vi "PID_controller_17.vi"() -> ()   [LabVIEW 2011]
panel:
  in  "Local":bool
  in  "Hold":bool
  out "tune_Method":u16(ring) items=["Setpoint", "Angle"]
  in  "Method":u16(ring)=1 items=["Setpoint", "Angle"]
  in  "Setpoint":u16(ring)=2 items=["A", "B", "C", "D"]
  out "do_tune":bool
  in  "Tune":bool
  out "Tune Set Point (torr)":dbl format="%.2f"
  in  "stop":bool
  out "fit":cluster{"element":dbl, "Value":dbl}[](array[cluster])
  out "err_avg":dbl
  out "Setpoint":string
  in  "Ks":dbl
  out "dt(s)":dbl
  out "windup error":dbl
  out "tPrev":dbl
  out "target value":dbl
  out "error(t-t0)":cluster{dbl, "Value":dbl}[](array[cluster])
  out "error":dbl
  out "tStart(s)":dbl
  out "S00":dbl
  out "S10":dbl
  out "S20":dbl
  out "S11":dbl
  out "S01":dbl
  out "weight":dbl[](array[numeric])
  in  "# of points to watch":i32=60
  in  "tSmooth(s)":dbl=4.0
  out "t0":dbl
  out "error(t)":cluster{dbl, "Value":dbl}[](array[cluster])
  out "error out":errorcluster
  out "first":bool=TRUE
  out "XY Graph":T1(graph)
  out "current value":dbl
  in  "Period (s)":dbl=1.0
  out "dValue":dbl
  out "derivative":dbl
  out "integral":dbl
  out "Angle (deg)":dbl format="%#.1f"
  in  "Kd":dbl=0.4
  in  "Ki":dbl
  in  "Kp":dbl=-0.1
  out "Current P (torr)":dbl format="%.2f"
  in  "Set Point (torr)":dbl format="%.2f"
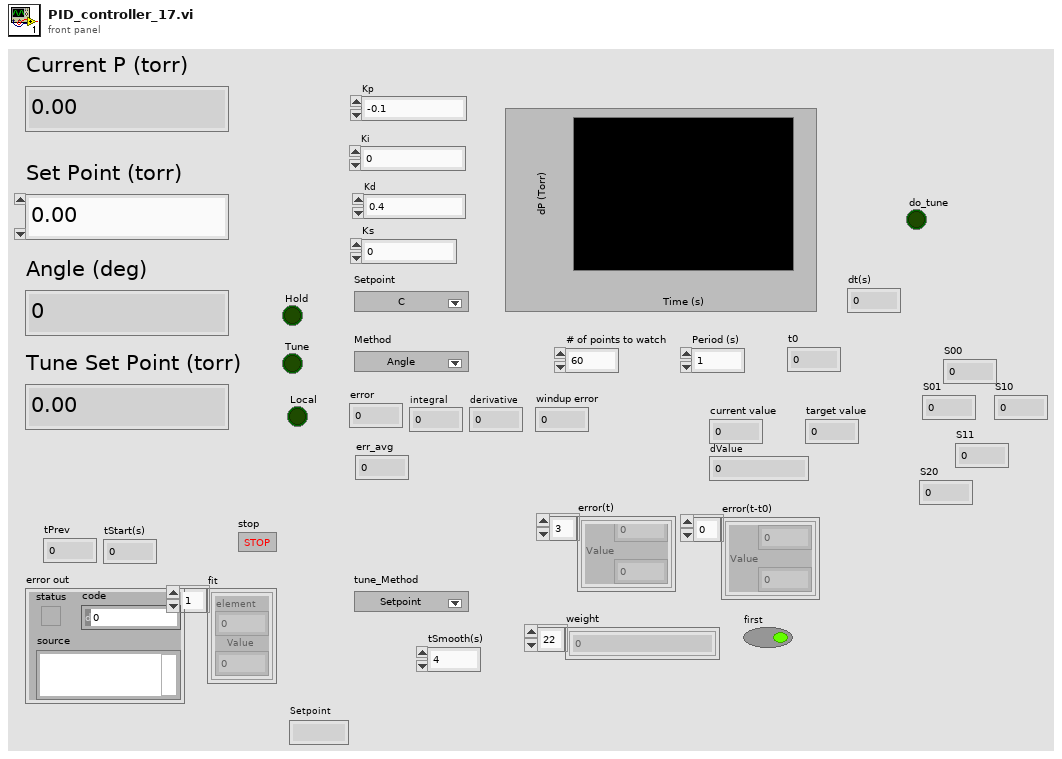
[diagram p1: front panel]
types:
  T1 = cluster{"Value":cluster{"element":dbl, "Value":dbl}[]}[]
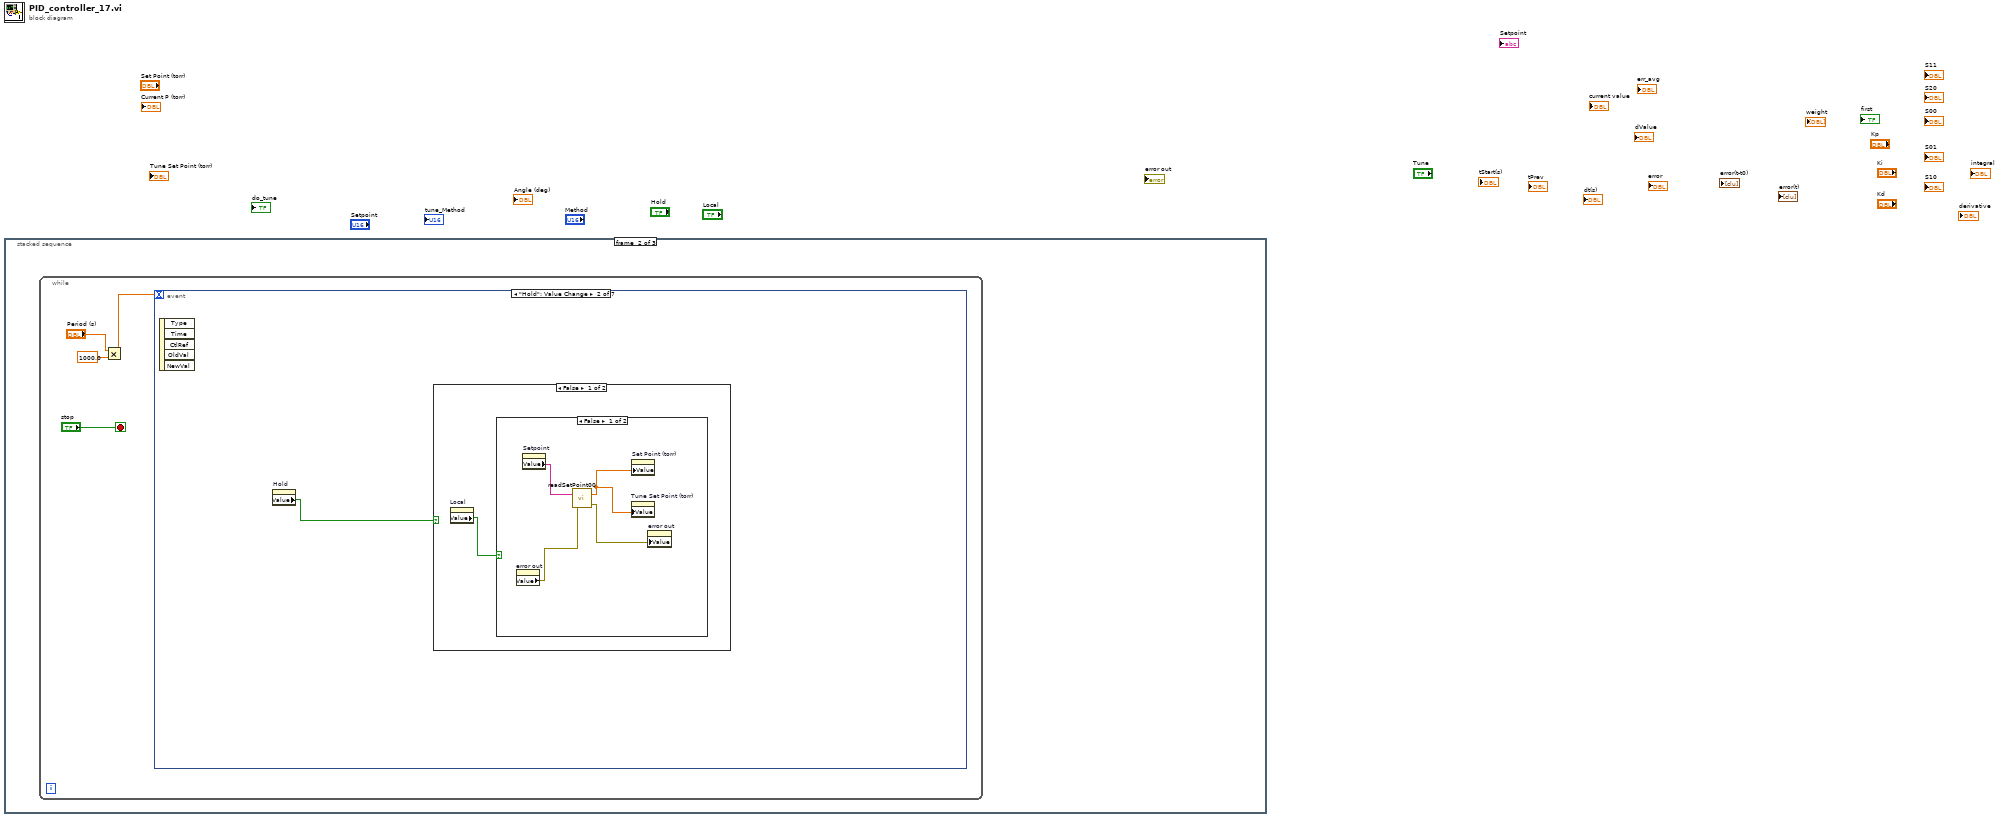
[diagram p0: block diagram]
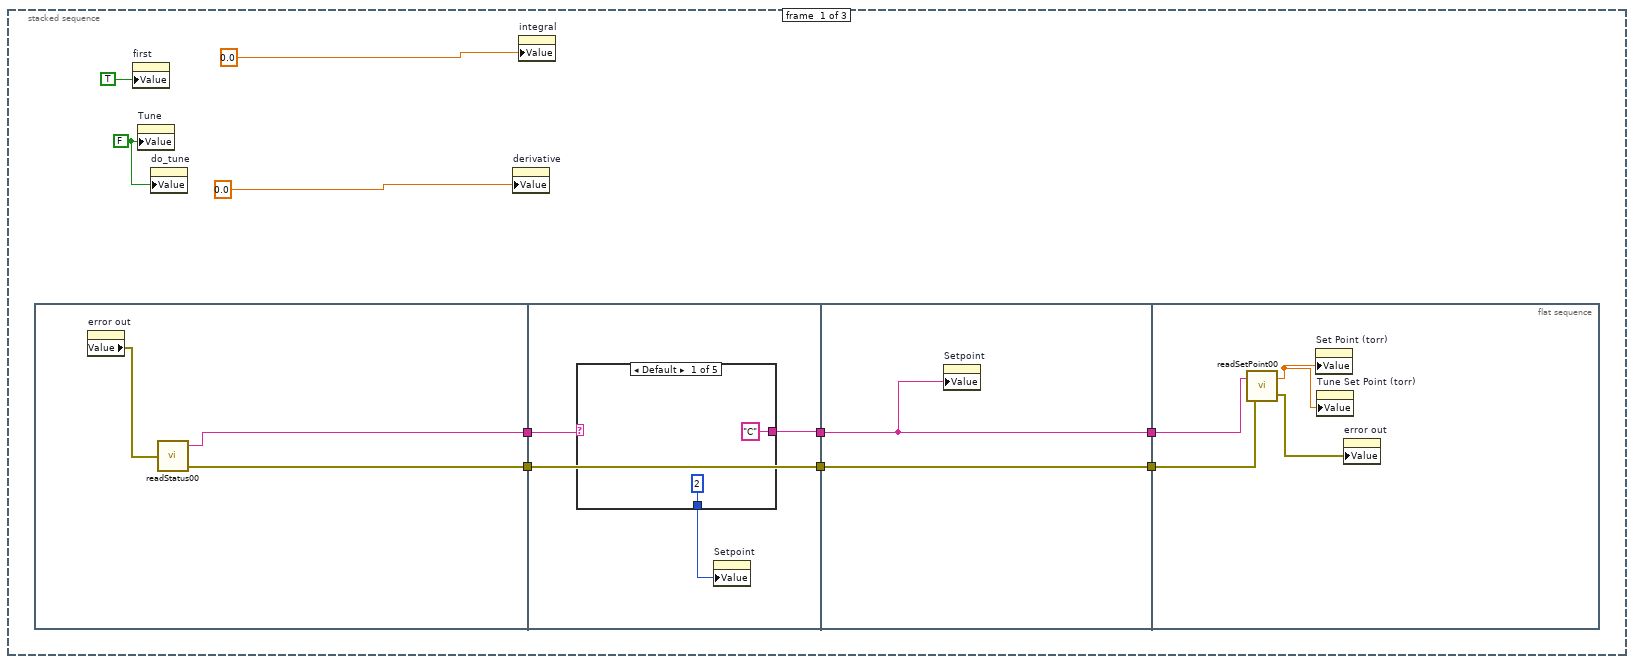
[diagram p2: hidden frame]
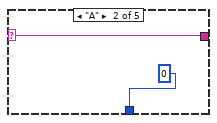
[diagram p3: hidden frame]
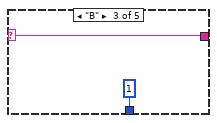
[diagram p4: hidden frame]
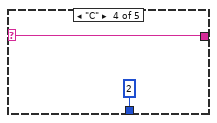
[diagram p5: hidden frame]
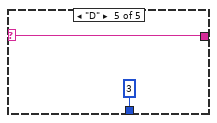
[diagram p6: hidden frame]
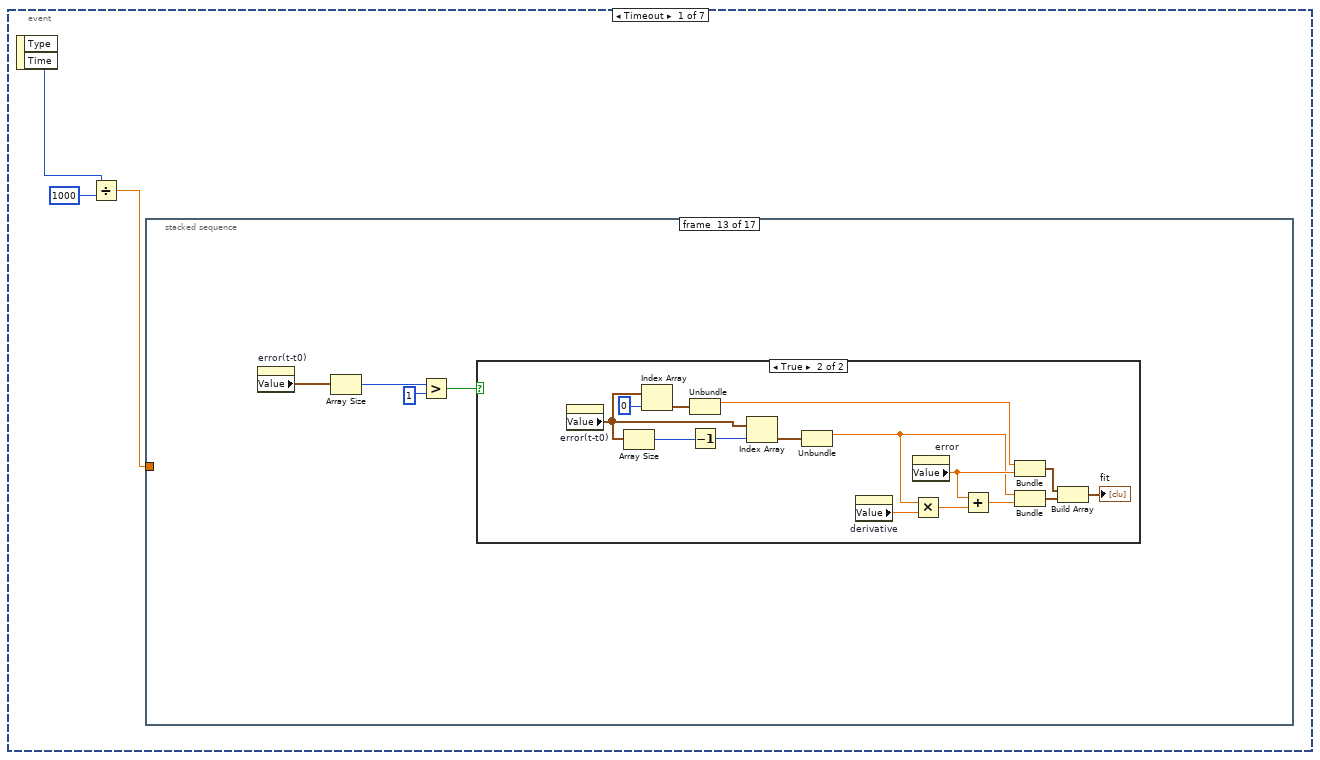
[diagram p7: hidden frame]
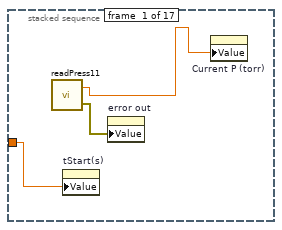
[diagram p8: hidden frame]
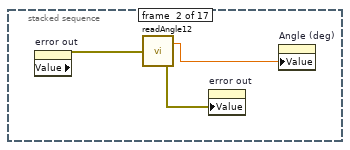
[diagram p9: hidden frame]
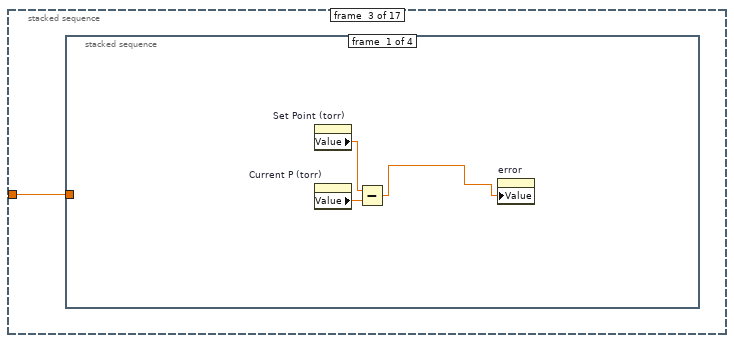
[diagram p10: hidden frame]
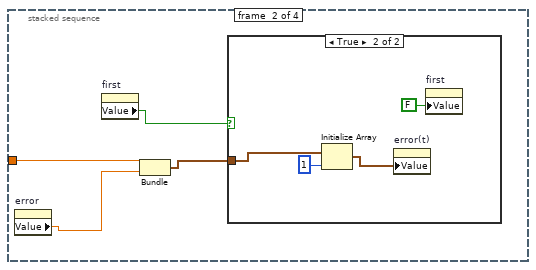
[diagram p11: hidden frame]
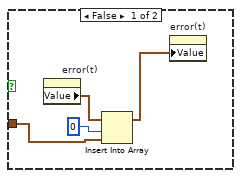
[diagram p12: hidden frame]
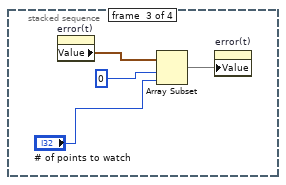
[diagram p13: hidden frame]
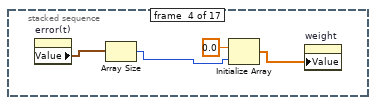
[diagram p15: hidden frame]
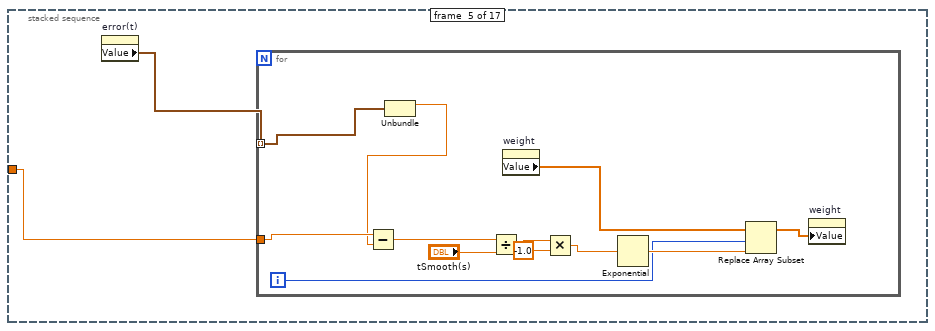
[diagram p16: hidden frame]
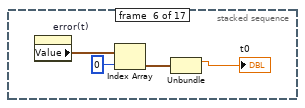
[diagram p17: hidden frame]
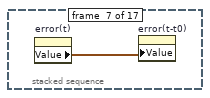
[diagram p18: hidden frame]
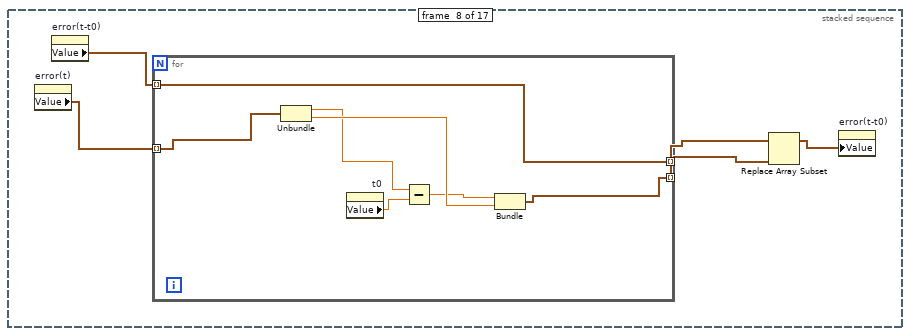
[diagram p19: hidden frame]
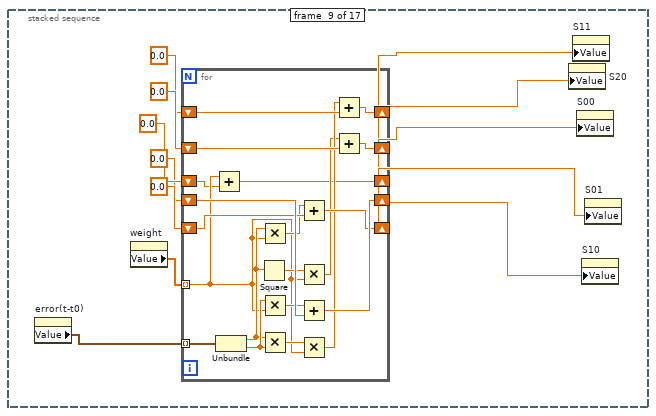
[diagram p20: hidden frame]
diagram:
  n1 = stacked-sequence {
    frame #0 {
      w7 = FALSE ("Tune")
      n2 = flat-sequence {
        tunnel: [w12] -> w6
        tunnel: [w11] -> w5
        tunnel: w6 -> [w16]
        tunnel: [w15] -> w4
        tunnel: w5 -> [w17]
        tunnel: [w17] -> w2
        tunnel: w4 -> [w28]
        tunnel: [w28] -> w3
        tunnel: w2 -> [w29]
        tunnel: [w29] -> w1
        tunnel: w3 -> [w33]
        tunnel: w1 -> [w32]
        frame #0 {
          n3 = property on="error out" class="Clust (strict)"() -> ("Value"=w13:errorcluster)  [unwired: 2 in, 2 out]
          n4 = call "readStatus00.vi"("error in"=w13) -> ("Setpoint"=w12:string, "error out"=w11:errorcluster)  [unwired: 1 out]
        }
        frame #1 {
          n5 = case shown="Default" w16 {
            selector: w16 -> [_ w21 w22 w24 w26]
            tunnel: ["C" w21 w22 w24 w26] -> w15
            tunnel: [u16 2 ("Ring") u16 0 ("Ring") u16 1 ("Ring") u16 2 ("Ring") u16 3 ("Ring")] -> w14
            frame Default {
            }
            frame "A" {
            }
            frame "B" {
            }
            frame "C" {
            }
            frame "D" {
            }
          }
          n6 = property on="Setpoint" class="Ring (strict)"("Value"=w14) -> ()  [unwired: 2 in, 2 out]
        }
        frame #2 {
          n7 = property on="Setpoint" class="Str"("Value"=w28) -> ()  [unwired: 2 in, 2 out]
        }
        frame #3 {
          n8 = call "readSetPoint00.vi"("error in"=w32, "Setpoint"=w33) -> ("error out"=w31:errorcluster, "P"=w30:dbl)
          n9 = property on="Set Point (torr)" class="DigNum (strict)"("Value"=w30) -> ()  [unwired: 2 in, 2 out]
          n10 = property on="Tune Set Point (torr)" class="DigNum (strict)"("Value"=w30) -> ()  [unwired: 2 in, 2 out]
          n11 = property on="error out" class="Clust (strict)"("Value"=w31) -> ()  [unwired: 2 in, 2 out]
        }
      }
      n12 = property on="first" class="Bool (strict)"("Value"=TRUE ("first")) -> ()  [unwired: 2 in, 2 out]
      n13 = property on="Tune" class="Bool (strict)"("Value"=w7) -> ()  [unwired: 2 in, 2 out]
      n14 = property on="do_tune" class="Bool (strict)"("Value"=w7) -> ()  [unwired: 2 in, 2 out]
      n15 = property on="derivative" class="DigNum (strict)"("Value"=0.0 ("derivative")) -> ()  [unwired: 2 in, 2 out]
      n16 = property on="integral" class="DigNum (strict)"("Value"=0.0 ("integral")) -> ()  [unwired: 2 in, 2 out]
    }
    frame #1 {
      n17 = while {
        stop <- "stop" stop-if-true
        n18 = Multiply(x="Period (s)", y=1000.0) -> (x*y=w35:dbl)
        n19 = event shown="[1] \"Hold\": Value Change" {
          selector: _ -> [_ _ _ _ _ _ _]
          dyn-events: _ -> [_ _ _ _ _ _ _]
          timeout: w35 -> [_ _ _ _ _ _ _]
          event Timeout {
            n20 = event-data() -> ("Time"=w40:u32)  [unwired: 1 in, 1 out]
            n21 = Divide(x=w40, y=u32 1000) -> (x/y=w38:dbl)
            n22 = stacked-sequence {
              tunnel: w38 -> [w41 _ w47 _ w71 _ _ _ _ _ _ _ _ _ _ _ _]
              frame #0 {
                n23 = call "readPress11.vi"() -> ("P"=w43:dbl, "error out"=w42:errorcluster)  [unwired: 1 in]
                n24 = property on="tStart(s)" class="DigNum (strict)"("Value"=w41) -> ()  [unwired: 2 in, 2 out]
                n25 = property on="error out" class="Clust (strict)"("Value"=w42) -> ()  [unwired: 2 in, 2 out]
                n26 = property on="Current P (torr)" class="DigNum (strict)"("Value"=w43) -> ()  [unwired: 2 in, 2 out]
              }
              frame #1 {
                n27 = property on="error out" class="Clust (strict)"() -> ("Value"=w45:errorcluster)  [unwired: 2 in, 2 out]
                n28 = call "readAngle12.vi"("error in"=w45) -> ("angle"=w46:dbl, "error out"=w44:errorcluster)
                n29 = property on="error out" class="Clust (strict)"("Value"=w44) -> ()  [unwired: 2 in, 2 out]
                n30 = property on="Angle (deg)" class="DigNum (strict)"("Value"=w46) -> ()  [unwired: 2 in, 2 out]
              }
              frame #2 {
                n31 = stacked-sequence {
                  tunnel: w47 -> [_ w53 _ _]
                  frame #0 {
                    n32 = property on="Set Point (torr)" class="DigNum (strict)"() -> ("Value"=w49:dbl)  [unwired: 2 in, 2 out]
                    n33 = property on="Current P (torr)" class="DigNum (strict)"() -> ("Value"=w50:dbl)  [unwired: 2 in, 2 out]
                    n34 = Subtract(x=w49, y=w50) -> (x-y=w48:dbl)
                    n35 = property on="error" class="DigNum (strict)"("Value"=w48) -> ()  [unwired: 2 in, 2 out]
                  }
                  frame #1 {
                    n36 = property on="error" class="DigNum (strict)"() -> ("Value"=w51:dbl)  [unwired: 2 in, 2 out]
                    n37 = property on="first" class="Bool (strict)"() -> ("Value"=w54:bool)  [unwired: 2 in, 2 out]
                    n38 = Bundle(w53, "Value"=w51) -> (w52:cluster{dbl, "Value":dbl})  [unwired: 1 in]
                    n39 = case shown="True" w54 {
                      tunnel: w52 -> [w56 w61]
                      frame False {
                        n40 = property on="error(t)" class="Arr (strict)"() -> ("Value"=w57:cluster{dbl, "Value":dbl}[])  [unwired: 2 in, 2 out]
                        n41 = Insert Into Array(array=w57, index=0, new element=w56) -> (w55:cluster{dbl, "Value":dbl}[])
                        n42 = property on="error(t)" class="Arr (strict)"("Value"=w55) -> ()  [unwired: 2 in, 2 out]
                      }
                      frame True {
                        n43 = Initialize Array(w61, 1 ("dimension size")) -> (w59:cluster{dbl, "Value":dbl}[])
                        n44 = property on="error(t)" class="Arr (strict)"("Value"=w59) -> ()  [unwired: 2 in, 2 out]
                        n45 = property on="first" class="Bool (strict)"("Value"=FALSE ("first")) -> ()  [unwired: 2 in, 2 out]
                      }
                    }
                  }
                  frame #2 {
                    n46 = property on="error(t)" class="Arr (strict)"() -> ("Value"=w64:cluster{dbl, "Value":dbl}[])  [unwired: 2 in, 2 out]
                    n47 = Array Subset(array=w64, index=0, length="# of points to watch") -> (w66:cluster{dbl, "Value":dbl}[])
                    n48 = property on="error(t)" class="Arr (strict)"("Value"=w66) -> ()  [unwired: 2 in, 2 out]
                  }
                  frame #3 {
                  }
                }
              }
              frame #3 {
                n49 = property on="error(t)" class="Arr (strict)"() -> ("Value"=w67:cluster{dbl, "Value":dbl}[])  [unwired: 2 in, 2 out]
                n50 = Array Size(array=w67) -> (size(s)=w69:i32)
                n51 = Initialize Array(0.0 ("element"), w69) -> (w70:dbl[])
                n52 = property on="weight" class="Arr (strict)"("Value"=w70) -> ()  [unwired: 2 in, 2 out]
              }
              frame #4 {
                n53 = property on="error(t)" class="Arr (strict)"() -> ("Value"=w72:cluster{dbl, "Value":dbl}[])  [unwired: 2 in, 2 out]
                n54 = for {
                  tunnel: w72 -> [w84] mode=indexing
                  tunnel: w71 -> [w83]
                  i -> [w79]
                  n55 = Unbundle(w84) -> (w82:dbl)  [unwired: 1 out]
                  n56 = Subtract(x=w83, y=w82) -> (x-y=w77:dbl)
                  n57 = Divide(x=w77, y="tSmooth(s)") -> (x/y=w75:dbl)
                  n58 = property on="weight" class="Arr (strict)"() -> ("Value"=w80:dbl[])  [unwired: 2 in, 2 out]
                  n59 = Multiply(x=w75, y=-1.0) -> (x*y=w73:dbl)
                  n60 = Exponential(1:w73) -> (0:w81:dbl)
                  n61 = Replace Array Subset(array=w80, new element=w81, index=w79) -> (w78:dbl[])
                  n62 = property on="weight" class="Arr (strict)"("Value"=w78) -> ()  [unwired: 2 in, 2 out]
                }
              }
              frame #5 {
                n63 = property on="error(t)" class="Arr (strict)"() -> ("Value"=w85:cluster{dbl, "Value":dbl}[])  [unwired: 2 in, 2 out]
                n64 = Index Array(array=w85, index=0) -> (element=w87:cluster{dbl, "Value":dbl})
                n65 = Unbundle(w87) -> (→"t0":dbl)  [unwired: 1 out]
              }
              frame #6 {
                n66 = property on="error(t)" class="Arr (strict)"() -> ("Value"=w89:cluster{dbl, "Value":dbl}[])  [unwired: 2 in, 2 out]
                n67 = property on="error(t-t0)" class="Arr (strict)"("Value"=w89) -> ()  [unwired: 2 in, 2 out]
              }
              frame #7 {
                n68 = property on="error(t)" class="Arr (strict)"() -> ("Value"=w90:cluster{dbl, "Value":dbl}[])  [unwired: 2 in, 2 out]
                n69 = property on="error(t-t0)" class="Arr (strict)"() -> ("Value"=w92:cluster{dbl, "Value":dbl}[])  [unwired: 2 in, 2 out]
                n70 = for {
                  tunnel: w90 -> [w97] mode=indexing
                  tunnel: [w96] -> w91 mode=indexing
                  tunnel: w92 -> [w95] mode=indexing
                  tunnel: [w95] -> w93 mode=indexing
                  n71 = Unbundle(w97) -> (w98:dbl, "Value"=w100:dbl)
                  n72 = property on="t0" class="DigNum (strict)"() -> ("Value"=w101:dbl)  [unwired: 2 in, 2 out]
                  n73 = Subtract(x=w98, y=w101) -> (x-y=w99:dbl)
                  n74 = Bundle(w99, "Value"=w100) -> (w96:cluster{dbl, "Value":dbl})  [unwired: 1 in]
                }
                n75 = Replace Array Subset(array=w93, new element=w91) -> (w94:cluster{dbl, "Value":dbl}[])  [unwired: 1 in]
                n76 = property on="error(t-t0)" class="Arr (strict)"("Value"=w94) -> ()  [unwired: 2 in, 2 out]
              }
              frame #8 {
                n77 = property on="error(t-t0)" class="Arr (strict)"() -> ("Value"=w113:cluster{dbl, "Value":dbl}[])  [unwired: 2 in, 2 out]
                n78 = property on="weight" class="Arr (strict)"() -> ("Value"=w106:dbl[])  [unwired: 2 in, 2 out]
                n79 = for {
                  tunnel: w113 -> [w129] mode=indexing
                  shift-right: [w130] -> w111
                  shift-left: 0.0 -> [w133]
                  shift-right: [w126] -> w108
                  shift-left: 0.0 -> [w132]
                  shift-right: [w125] -> w109
                  shift-left: 0.0 -> [w131]
                  shift-right: [w127] -> w112
                  shift-left: 0.0 -> [w128]
                  tunnel: w106 -> [w116] mode=indexing
                  shift-right: [w114] -> w110
                  shift-left: 0.0 -> [w115]
                  n80 = Add(x=w116, y=w115) -> (x+y=w114:dbl)
                  n81 = Unbundle(w129) -> (w118:dbl, "Value"=w124:dbl)
                  n82 = Square(x=w118) -> (x^2=w120:dbl)
                  n83 = Multiply(x=w118, y=w116) -> (x*y=w117:dbl)
                  n84 = Multiply(x=w124, y=w116) -> (x*y=w123:dbl)
                  n85 = Multiply(x=w118, y=w124) -> (x*y=w122:dbl)
                  n86 = Add(x=w117, y=w128) -> (x+y=w127:dbl)
                  n87 = Multiply(x=w120, y=w116) -> (x*y=w119:dbl)
                  n88 = Add(x=w123, y=w133) -> (x+y=w130:dbl)
                  n89 = Multiply(x=w122, y=w116) -> (x*y=w121:dbl)
                  n90 = Add(x=w121, y=w132) -> (x+y=w126:dbl)
                  n91 = Add(x=w119, y=w131) -> (x+y=w125:dbl)
                }
                n92 = property on="S20" class="DigNum (strict)"("Value"=w109) -> ()  [unwired: 2 in, 2 out]
                n93 = property on="S11" class="DigNum (strict)"("Value"=w108) -> ()  [unwired: 2 in, 2 out]
                n94 = property on="S00" class="DigNum (strict)"("Value"=w110) -> ()  [unwired: 2 in, 2 out]
                n95 = property on="S10" class="DigNum (strict)"("Value"=w112) -> ()  [unwired: 2 in, 2 out]
                n96 = property on="S01" class="DigNum (strict)"("Value"=w111) -> ()  [unwired: 2 in, 2 out]
              }
              frame #9 {
                n97 = property on="S00" class="DigNum (strict)"() -> ("Value"=w135:dbl)  [unwired: 2 in, 2 out]
                n98 = Greater Than 0?(x=w135) -> (x > 0?=w134:bool)
                n99 = case shown="True" w134 {
                  tunnel: w135 -> [_ w144]
                  frame False {
                    n100 = property on="derivative" class="DigNum (strict)"("Value"=0.0 ("derivative")) -> ()  [unwired: 2 in, 2 out]
                  }
                  frame True {
                    n101 = property on="S11" class="DigNum (strict)"() -> ("Value"=w146:dbl)  [unwired: 2 in, 2 out]
                    n102 = property on="S20" class="DigNum (strict)"() -> ("Value"=w145:dbl)  [unwired: 2 in, 2 out]
                    n103 = property on="S01" class="DigNum (strict)"() -> ("Value"=w143:dbl)  [unwired: 2 in, 2 out]
                    n104 = property on="S10" class="DigNum (strict)"() -> ("Value"=w147:dbl)  [unwired: 2 in, 2 out]
                    n105 = Multiply(x=w144, y=w146) -> (x*y=w152:dbl)
                    n106 = Multiply(x=w144, y=w145) -> (x*y=w150:dbl)
                    n107 = Multiply(x=w143, y=w147) -> (x*y=w151:dbl)
                    n108 = Square(x=w147) -> (x^2=w149:dbl)
                    n109 = Subtract(x=w152, y=w151) -> (x-y=w148:dbl)
                    n110 = Subtract(x=w150, y=w149) -> (x-y=w142:dbl)
                    n111 = Divide(x=w148, y=w142) -> (x/y=w138:dbl)
                    n112 = Greater?(x=w142, y=1e-07) -> (0:w140:bool)
                    n113 = Select(t=w138, s=w140, f=0.0) -> (s? t:f=w139:dbl)
                    n114 = property on="derivative" class="DigNum (strict)"("Value"=w139) -> ()  [unwired: 2 in, 2 out]
                  }
                }
              }
              frame #10 {
                n115 = property on="S00" class="DigNum (strict)"() -> ("Value"=w154:dbl)  [unwired: 2 in, 2 out]
                n116 = Greater Than 0?(x=w154) -> (x > 0?=w153:bool)
                n117 = case shown="True" w153 {
                  tunnel: w154 -> [_ w157]
                  frame False {
                    n118 = property on="err_avg" class="DigNum (strict)"("Value"=0.0 ("Pavg")) -> ()  [unwired: 2 in, 2 out]
                  }
                  frame True {
                    n119 = property on="S01" class="DigNum (strict)"() -> ("Value"=w158:dbl)  [unwired: 2 in, 2 out]
                    n120 = property on="S20" class="DigNum (strict)"() -> ("Value"=w161:dbl)  [unwired: 2 in, 2 out]
                    n121 = property on="S11" class="DigNum (strict)"() -> ("Value"=w159:dbl)  [unwired: 2 in, 2 out]
                    n122 = property on="S11" class="DigNum (strict)"() -> ("Value"=w160:dbl)  [unwired: 2 in, 2 out]
                    n123 = Multiply(x=w158, y=w161) -> (x*y=w166:dbl)
                    n124 = Multiply(x=w157, y=w161) -> (x*y=w163:dbl)
                    n125 = Multiply(x=w160, y=w159) -> (x*y=w167:dbl)
                    n126 = Square(x=w160) -> (x^2=w164:dbl)
                    n127 = Subtract(x=w166, y=w167) -> (x-y=w162:dbl)
                    n128 = Subtract(x=w163, y=w164) -> (x-y=w165:dbl)
                    n129 = Divide(x=w162, y=w165) -> (x/y=w156:dbl)
                    n130 = property on="err_avg" class="DigNum (strict)"("Value"=w156) -> ()  [unwired: 2 in, 2 out]
                  }
                }
              }
              frame #11 {
                n131 = property on="tStart(s)" class="DigNum (strict)"() -> ("Value"=w168:dbl)  [unwired: 2 in, 2 out]
                n132 = property on="tPrev" class="DigNum (strict)"("Value"=w168) -> ()  [unwired: 2 in, 2 out]
              }
              frame #12 {
                n133 = property on="error(t-t0)" class="Arr (strict)"() -> ("Value"=w169:cluster{dbl, "Value":dbl}[])  [unwired: 2 in, 2 out]
                n134 = Array Size(array=w169) -> (size(s)=w170:i32)
                n135 = Greater?(x=w170, y=1) -> (0:w172:bool)
                n136 = case shown="True" w172 {
                  frame False {
                  }
                  frame True {
                    n137 = property on="error(t-t0)" class="Arr (strict)"() -> ("Value"=w176:cluster{dbl, "Value":dbl}[])  [unwired: 2 in, 2 out]
                    n138 = Array Size(array=w176) -> (size(s)=w186:i32)
                    n139 = Index Array(array=w176, index=0) -> (element=w184:cluster{dbl, "Value":dbl})
                    n140 = Unbundle(w184) -> (w179:dbl)  [unwired: 1 out]
                    n141 = Decrement(x=w186) -> (x-1=w185:i32)
                    n142 = Index Array(array=w176, index=w185) -> (element=w183:cluster{dbl, "Value":dbl})
                    n143 = Unbundle(w183) -> (w177:dbl)  [unwired: 1 out]
                    n144 = property on="derivative" class="DigNum (strict)"() -> ("Value"=w182:dbl)  [unwired: 2 in, 2 out]
                    n145 = property on="error" class="DigNum (strict)"() -> ("Value"=w180:dbl)  [unwired: 2 in, 2 out]
                    n146 = Multiply(x=w177, y=w182) -> (x*y=w181:dbl)
                    n147 = Add(x=w180, y=w181) -> (x+y=w178:dbl)
                    n148 = Bundle(w179, "Value"=w180) -> (w175:cluster{dbl, "Value":dbl})  [unwired: 1 in]
                    n149 = Bundle(w177, w178) -> (w174:cluster{dbl, dbl})  [unwired: 1 in]
                    n150 = Build Array(w175, w174) -> (→"fit":cluster{dbl, "Value":dbl}[])
                  }
                }
              }
              frame #13 {
                n151 = property on="error" class="DigNum (strict)"() -> ("Value"=w190:dbl)  [unwired: 2 in, 2 out]
                n152 = property on="tPrev" class="DigNum (strict)"() -> ("Value"=w189:dbl)  [unwired: 2 in, 2 out]
                n153 = property on="tStart(s)" class="DigNum (strict)"() -> ("Value"=w188:dbl)  [unwired: 2 in, 2 out]
                n154 = Subtract(x=w188, y=w189) -> (x-y=w194:dbl)
                n155 = property on="dt(s)" class="DigNum (strict)"("Value"=w194) -> ()  [unwired: 2 in, 2 out]
                n156 = property on="integral" class="DigNum (strict)"() -> ("Value"=w192:dbl)  [unwired: 2 in, 2 out]
                n157 = Multiply(x=w190, y=w194) -> (x*y=w191:dbl)
                n158 = Add(x=w191, y=w192) -> (x+y=w193:dbl)
                n159 = property on="integral" class="DigNum (strict)"("Value"=w193) -> ()  [unwired: 2 in, 2 out]
              }
              frame #14 {
                n160 = property on="error" class="DigNum (strict)"() -> ("Value"=w207:dbl)  [unwired: 2 in, 2 out]
                n161 = property on="tune_Method" class="Ring (strict)"() -> ("Value"=w197:u16)  [unwired: 2 in, 2 out]
                n162 = property on="Kp" class="DigNum (strict)"() -> ("Value"=w196:dbl)  [unwired: 2 in, 2 out]
                n163 = property on="integral" class="DigNum (strict)"() -> ("Value"=w199:dbl)  [unwired: 2 in, 2 out]
                n164 = property on="derivative" class="DigNum (strict)"() -> ("Value"=w201:dbl)  [unwired: 2 in, 2 out]
                n165 = property on="Ki" class="DigNum (strict)"() -> ("Value"=w198:dbl)  [unwired: 2 in, 2 out]
                n166 = property on="Kd" class="DigNum (strict)"() -> ("Value"=w200:dbl)  [unwired: 2 in, 2 out]
                n167 = case shown="0, Default" w197 {
                  tunnel: w196 -> [w208 w211]
                  tunnel: [w208 w209] -> w195
                  frame 0, Default {
                  }
                  frame 1 {
                    n168 = Multiply(x=w211, y=-1.0) -> (x*y=w209:dbl)
                  }
                }
                n169 = Multiply(x=w200, y=w201) -> (x*y=w204:dbl)
                n170 = Multiply(x=w198, y=w199) -> (x*y=w203:dbl)
                n171 = Multiply(x=w195, y=w207) -> (x*y=w202:dbl)
                n172 = Add(x=w202, y=w203) -> (x+y=w205:dbl)
                n173 = Add(x=w205, y=w204) -> (x+y=w206:dbl)
                n174 = property on="dValue" class="DigNum (strict)"("Value"=w206) -> ()  [unwired: 2 in, 2 out]
              }
              frame #15 {
                n175 = property on="do_tune" class="Bool (strict)"() -> ("Value"=w212:bool)  [unwired: 2 in, 2 out]
                n176 = case shown="True" w212 {
                  frame False {
                  }
                  frame True {
                    w225 = 90.0 ("y")
                    n177 = property on="dValue" class="DigNum (strict)"() -> ("Value"=w230:dbl)  [unwired: 2 in, 2 out]
                    n178 = property on="current value" class="DigNum (strict)"() -> ("Value"=w231:dbl)  [unwired: 2 in, 2 out]
                    n179 = Add(x=w231, y=w230) -> (x+y=w217:dbl)
                    "target value" <- w217
                    n180 = Less Than 0?(x=w217) -> (x < 0?=w229:bool)
                    n181 = Select(t=0.0, s=w229, f=w217) -> (s? t:f=w226:dbl)
                    n182 = property on="error out" class="Clust (strict)"() -> ("Value"=w215:errorcluster)  [unwired: 2 in, 2 out]
                    n183 = Greater?(x=w226, y=w225) -> (0:w227:bool)
                    n184 = Select(t=w225, s=w227, f=w226) -> (s? t:f=w214:dbl)
                    n185 = Subtract(x=w214, y=w217) -> (x-y=w224:dbl)
                    "windup error" <- w224
                    n186 = property on="dt(s)" class="DigNum (strict)"() -> ("Value"=w223:dbl)  [unwired: 2 in, 2 out]
                    n187 = property on="current value" class="DigNum (strict)"("Value"=w214) -> ()  [unwired: 2 in, 2 out]
                    n188 = property on="tune_Method" class="Ring (strict)"() -> ("Value"=w216:u16)  [unwired: 2 in, 2 out]
                    n189 = Multiply(x=w224, y=w223) -> (x*y=w222:dbl)
                    n190 = property on="integral" class="DigNum (strict)"() -> ("Value"=w219:dbl)  [unwired: 2 in, 2 out]
                    n191 = Multiply(x="Ks", y=w222) -> (x*y=w220:dbl)
                    n192 = case shown="0, Default" w216 {
                      tunnel: w215 -> [w235 w238]
                      tunnel: w214 -> [w234 w237]
                      tunnel: [w232 w236] -> w213
                      frame 0, Default {
                        n193 = property on="Setpoint" class="Str"() -> ("Value"=w233:string)  [unwired: 2 in, 2 out]
                        n194 = property on="Tune Set Point (torr)" class="DigNum (strict)"("Value"=w234) -> ()  [unwired: 2 in, 2 out]
                        n195 = call "writeSetPoint_00.vi"("error in"=w235, "P (Torr)"=w234, "Setpoint"=w233) -> ("error out"=w232:errorcluster)
                      }
                      frame 1 {
                        n196 = call "setAngle_00.vi"("error in (no error)"=w238, "Angle (deg)"=w237) -> ("error out"=w236:errorcluster)
                      }
                    }
                    n197 = Add(x=w220, y=w219) -> (x+y=w218:dbl)
                    n198 = property on="integral" class="DigNum (strict)"("Value"=w218) -> ()  [unwired: 2 in, 2 out]
                    n199 = property on="error out" class="Clust (strict)"("Value"=w213) -> ()  [unwired: 2 in, 2 out]
                  }
                }
              }
              frame #16 {
                n200 = property on="fit" class="Arr (strict)"() -> ("Value"=w241:cluster{"element":dbl, "Value":dbl}[])  [unwired: 2 in, 2 out]
                n201 = property on="error(t-t0)" class="Arr (strict)"() -> ("Value"=w240:cluster{dbl, "Value":dbl}[])  [unwired: 2 in, 2 out]
                n202 = Build Cluster Array(w240, w241) -> (→"XY Graph":T1)
              }
            }
          }
          event "Hold": Value Change {
            n203 = event-data() -> ()  [unwired: 1 in, 5 out]
            n204 = property on="Hold" class="Bool (strict)"() -> ("Value"=w242:bool)  [unwired: 2 in, 2 out]
            n205 = case shown="False" w242 {
              frame False {
                n206 = property on="Local" class="Bool (strict)"() -> ("Value"=w243:bool)  [unwired: 2 in, 2 out]
                n207 = case shown="False" w243 {
                  frame False {
                    n208 = property on="error out" class="Clust (strict)"() -> ("Value"=w247:errorcluster)  [unwired: 2 in, 2 out]
                    n209 = property on="Setpoint" class="Str"() -> ("Value"=w244:string)  [unwired: 2 in, 2 out]
                    n210 = call "readSetPoint00.vi"("error in"=w247, "Setpoint"=w244) -> ("error out"=w246:errorcluster, "P"=w245:dbl)
                    n211 = property on="Tune Set Point (torr)" class="DigNum (strict)"("Value"=w245) -> ()  [unwired: 2 in, 2 out]
                    n212 = property on="Set Point (torr)" class="DigNum (strict)"("Value"=w245) -> ()  [unwired: 2 in, 2 out]
                    n213 = property on="error out" class="Clust (strict)"("Value"=w246) -> ()  [unwired: 2 in, 2 out]
                  }
                  frame True {
                  }
                }
              }
              frame True {
                n214 = property on="error out" class="Clust (strict)"() -> ("Value"=w251:errorcluster)  [unwired: 2 in, 2 out]
                n215 = property on="Tune" class="Bool (strict)"("Value"=FALSE ("Tune")) -> ()  [unwired: 2 in, 2 out]
                n216 = property on="Local" class="Bool (strict)"("Value"=FALSE ("Local")) -> ()  [unwired: 2 in, 2 out]
                n217 = call "WriteAdaptorr03.vi"("error in (no error)"=w251, "string to write"="H") -> ("error out"=w250:errorcluster)
                n218 = property on="error out" class="Clust (strict)"("Value"=w250) -> ()  [unwired: 2 in, 2 out]
              }
            }
          }
          event "Local": Value Change {
            n219 = event-data() -> ()  [unwired: 1 in, 5 out]
            n220 = property on="Local" class="Bool (strict)"() -> ("Value"=w253:bool)  [unwired: 2 in, 2 out]
            n221 = case shown="True" w253 {
              frame False {
                n222 = property on="error out" class="Clust (strict)"() -> ("Value"=w256:errorcluster)  [unwired: 2 in, 2 out]
                n223 = call "WriteAdaptorr03.vi"("error in (no error)"=w256, "string to write"="H") -> ("error out"=w255:errorcluster)
                n224 = property on="Hold" class="Bool (strict)"("Value"=TRUE ("Hold")) -> ()  [unwired: 2 in, 2 out]
                n225 = property on="error out" class="Clust (strict)"("Value"=w255) -> ()  [unwired: 2 in, 2 out]
              }
              frame True {
                n226 = property on="error out" class="Clust (strict)"() -> ("Value"=w260:errorcluster)  [unwired: 2 in, 2 out]
                n227 = call "WriteAdaptorr03.vi"("error in (no error)"=w260, "string to write"="D5") -> ("error out"=w261:errorcluster)
                n228 = property on="Hold" class="Bool (strict)"("Value"=FALSE ("Hold")) -> ()  [unwired: 2 in, 2 out]
                n229 = property on="error out" class="Clust (strict)"("Value"=w261) -> ()  [unwired: 2 in, 2 out]
              }
            }
          }
          event "Tune": Value Change {
            n230 = event-data() -> ()  [unwired: 1 in, 5 out]
            n231 = property on="Tune" class="Bool (strict)"() -> ("Value"=w262:bool)  [unwired: 2 in, 2 out]
            n232 = property on="do_tune" class="Bool (strict)"("Value"=w262) -> ()  [unwired: 2 in, 2 out]
            n233 = case shown="False" w262 {
              frame False {
                n234 = property on="tune_Method" class="Ring (strict)"() -> ("Value"=w263:u16)  [unwired: 2 in, 2 out]
                n235 = case shown="0, Default" w263 {
                  frame 0, Default {
                    n236 = property on="Set Point (torr)" class="DigNum (strict)"() -> ("Value"=w266:dbl)  [unwired: 2 in, 2 out]
                    n237 = property on="Setpoint" class="Str"() -> ("Value"=w267:string)  [unwired: 2 in, 2 out]
                    n238 = property on="error out" class="Clust (strict)"() -> ("Value"=w265:errorcluster)  [unwired: 2 in, 2 out]
                    n239 = call "writeSetPoint_00.vi"("error in"=w265, "P (Torr)"=w266, "Setpoint"=w267) -> ("error out"=w264:errorcluster)
                    n240 = property on="error out" class="Clust (strict)"("Value"=w264) -> ()  [unwired: 2 in, 2 out]
                  }
                  frame 1 {
                    n241 = flat-sequence {
                      frame #0 {
                        n242 = call "WriteAdaptorr03.vi"("string to write"="D5") -> ()  [unwired: 1 in, 1 out]
                      }
                      frame #1 {
                        n243 = property on="Setpoint" class="Str"() -> ("Value"=w270:string)  [unwired: 2 in, 2 out]
                        n244 = Concatenate Strings("Press ", w270, " on AdapTorr") -> (w269:string)
                        n245 = One Button Dialog(message=w269) -> ()  [unwired: 1 in, 1 out]
                      }
                    }
                  }
                }
              }
              frame True {
                n246 = property on="error out" class="Clust (strict)"() -> ("Value"=w275:errorcluster)  [unwired: 2 in, 2 out]
                n247 = property on="Setpoint" class="Str"() -> ("Value"=w274:string)  [unwired: 2 in, 2 out]
                n248 = call "readSetPoint00.vi"("error in"=w275, "Setpoint"=w274) -> ("error out"=w276:errorcluster, "P"=w273:dbl)
                n249 = property on="Tune Set Point (torr)" class="DigNum (strict)"("Value"=w273) -> ()  [unwired: 2 in, 2 out]
                n250 = property on="Set Point (torr)" class="DigNum (strict)"("Value"=w273) -> ()  [unwired: 2 in, 2 out]
                n251 = property on="error out" class="Clust (strict)"("Value"=w276) -> ()  [unwired: 2 in, 2 out]
                n252 = property on="current value" class="DigNum (strict)"("Value"=w273) -> ()  [unwired: 2 in, 2 out]
              }
            }
          }
          event "Set Point (torr)": Value Change {
            n253 = event-data() -> ()  [unwired: 1 in, 5 out]
            n254 = property on="Set Point (torr)" class="DigNum (strict)"() -> ("Value"=w279:dbl)  [unwired: 2 in, 2 out]
            n255 = property on="Setpoint" class="Str"() -> ("Value"=w280:string)  [unwired: 2 in, 2 out]
            n256 = property on="error out" class="Clust (strict)"() -> ("Value"=w278:errorcluster)  [unwired: 2 in, 2 out]
            n257 = call "writeSetPoint_00.vi"("error in"=w278, "P (Torr)"=w279, "Setpoint"=w280) -> ("error out"=w277:errorcluster)
            n258 = property on="error out" class="Clust (strict)"("Value"=w277) -> ()  [unwired: 2 in, 2 out]
          }
          event "Setpoint": Value Change {
            n259 = event-data() -> ()  [unwired: 1 in, 5 out]
            n260 = property on="Setpoint" class="Ring (strict)"() -> ("Value"=w285:u16)  [unwired: 2 in, 2 out]
            n261 = case shown="3" w285 {
              tunnel: ["A" "B" "C" "D"] -> w281
              frame 0, Default {
              }
              frame 1 {
              }
              frame 2 {
              }
              frame 3 {
              }
            }
            n262 = property on="Setpoint" class="Str"("Value"=w281) -> ()  [unwired: 2 in, 2 out]
            n263 = property on="error out" class="Clust (strict)"() -> ("Value"=w282:errorcluster)  [unwired: 2 in, 2 out]
            n264 = call "readSetPoint00.vi"("error in"=w282, "Setpoint"=w281) -> ("error out"=w283:errorcluster, "P"=w284:dbl)
            n265 = property on="Set Point (torr)" class="DigNum (strict)"("Value"=w284) -> ()  [unwired: 2 in, 2 out]
            n266 = property on="Tune Set Point (torr)" class="DigNum (strict)"("Value"=w284) -> ()  [unwired: 2 in, 2 out]
            n267 = property on="error out" class="Clust (strict)"("Value"=w283) -> ()  [unwired: 2 in, 2 out]
          }
          event "Method": Value Change {
            n268 = event-data() -> ()  [unwired: 1 in, 5 out]
            n269 = property on="Method" class="Ring (strict)"() -> ("Value"=w290:u16)  [unwired: 2 in, 2 out]
            n270 = case shown="1" w290 {
              frame 0, Default {
              }
              frame 1 {
                n271 = property on="do_tune" class="Bool (strict)"() -> ("Value"=w291:bool)  [unwired: 2 in, 2 out]
                n272 = case shown="True" w291 {
                  frame False {
                  }
                  frame True {
                    n273 = flat-sequence {
                      frame #0 {
                        n274 = call "WriteAdaptorr03.vi"("string to write"="D5") -> ()  [unwired: 1 in, 1 out]
                      }
                      frame #1 {
                        n275 = property on="Setpoint" class="Str"() -> ("Value"=w294:string)  [unwired: 2 in, 2 out]
                        n276 = Concatenate Strings("Press ", w294, " on AdapTorr") -> (w293:string)
                        n277 = One Button Dialog(message=w293) -> ()  [unwired: 1 in, 1 out]
                      }
                    }
                  }
                }
              }
            }
            n278 = property on="tune_Method" class="Ring (strict)"("Value"=w290) -> ()  [unwired: 2 in, 2 out]
          }
        }
      }
    }
    frame #2 {
      n279 = property on="tune_Method" class="Ring (strict)"() -> ("Value"=w297:u16)  [unwired: 2 in, 2 out]
      n280 = case shown="1" w297 {
        frame 0, Default {
        }
        frame 1 {
          n281 = flat-sequence {
            frame #0 {
              n282 = property on="error out" class="Clust (strict)"() -> ("Value"=w299:errorcluster)  [unwired: 2 in, 2 out]
              n283 = call "setLocal_And_Hold_00.vi"("error in (no error)"=w299) -> ("error out"=w298:errorcluster)
              n284 = property on="error out" class="Clust (strict)"("Value"=w298) -> ()  [unwired: 2 in, 2 out]
            }
            frame #1 {
              n285 = property on="Setpoint" class="Str"() -> ("Value"=w301:string)  [unwired: 2 in, 2 out]
              n286 = Concatenate Strings("Press ", w301, " on AdapTorr") -> (w300:string)
              n287 = One Button Dialog(message=w300) -> ()  [unwired: 1 in, 1 out]
            }
          }
        }
      }
    }
  }
